vi "Percentage.vi"(1 "A":i32, 2 "B":i32) -> (0 "B/A (%)":dbl)   [LabVIEW 2023, in "VIA Results Handling.lvlib"]
doc: "Calculates the percentage of B / A"
uses:
  VIA Results Handling.lvlib
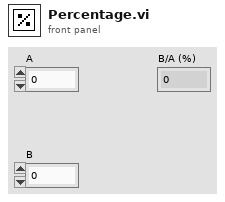
[diagram p1: front panel]
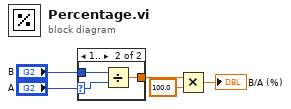
[diagram p0: block diagram]
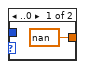
[diagram p2: hidden frame]
diagram:
  n1 = case shown="1.." "A" {
    selector: "A" -> [_ w9]
    tunnel: "B" -> [_ w8]
    tunnel: [nan w7] -> w3
    frame ..0 {
    }
    frame 1.. {
      n2 = Divide(x=w8, y=w9) -> (x/y=w7:dbl)
    }
  }
  n3 = Multiply(x=w3, y=100.0) -> (x*y=→"B/A (%)":dbl)
